vi "Insight LT.vi"(0 "Scroll Timing":i32=1500, 1 "ZONE \nCONFIGURATION":T1(ring), 2 "Digital Module":T2, 3 "Zone 4 Data":string[](array[string]), 4 "Zone 3 Data":string[](array[string]), 5 "Zone 2 Data":string[](array[string]), 6 "Zone 1 Data":string[](array[string])) -> ()   [LabVIEW 2012]
uses:
  <vilib>/Rock Robotics/SystemInterfaces/Typedef/FPGA_TypedefDigitalModule.ctl
panel:
  out "Zone 1 Index Count Line 2":i8
  out "Index Timer":dbl
  out "Zone 4 Index Count":i8
  out "Zone 3 Index Count":i8
  out "Zone 2 Index Count":i8
  out "Zone 1 Index Count":i8
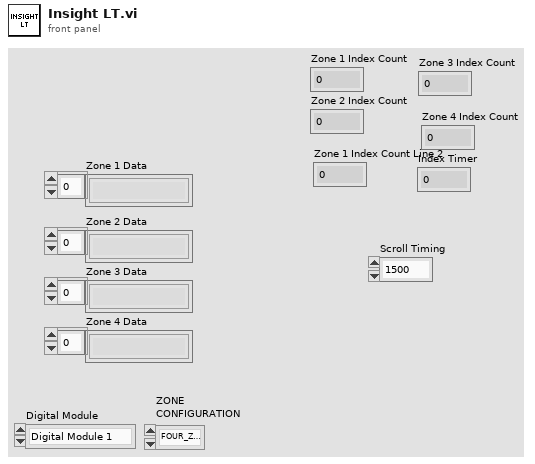
[diagram p1: front panel]
types:
  T1 = enum16{"FOUR_ZONES", "ONE_ZONE_TWO_LINES", "TWO_ZONES_ONE_LINE"}
  T2 = typedef "FPGA_TypedefDigitalModule.ctl" = enum16{"Digital Module 1", "Digital Module 2"}
  T3 = typedef "WPI_I2CDevRef.ctl" = cluster{"DevStatus":errorcluster, "Digital Module":T2, "Device Address":u8}
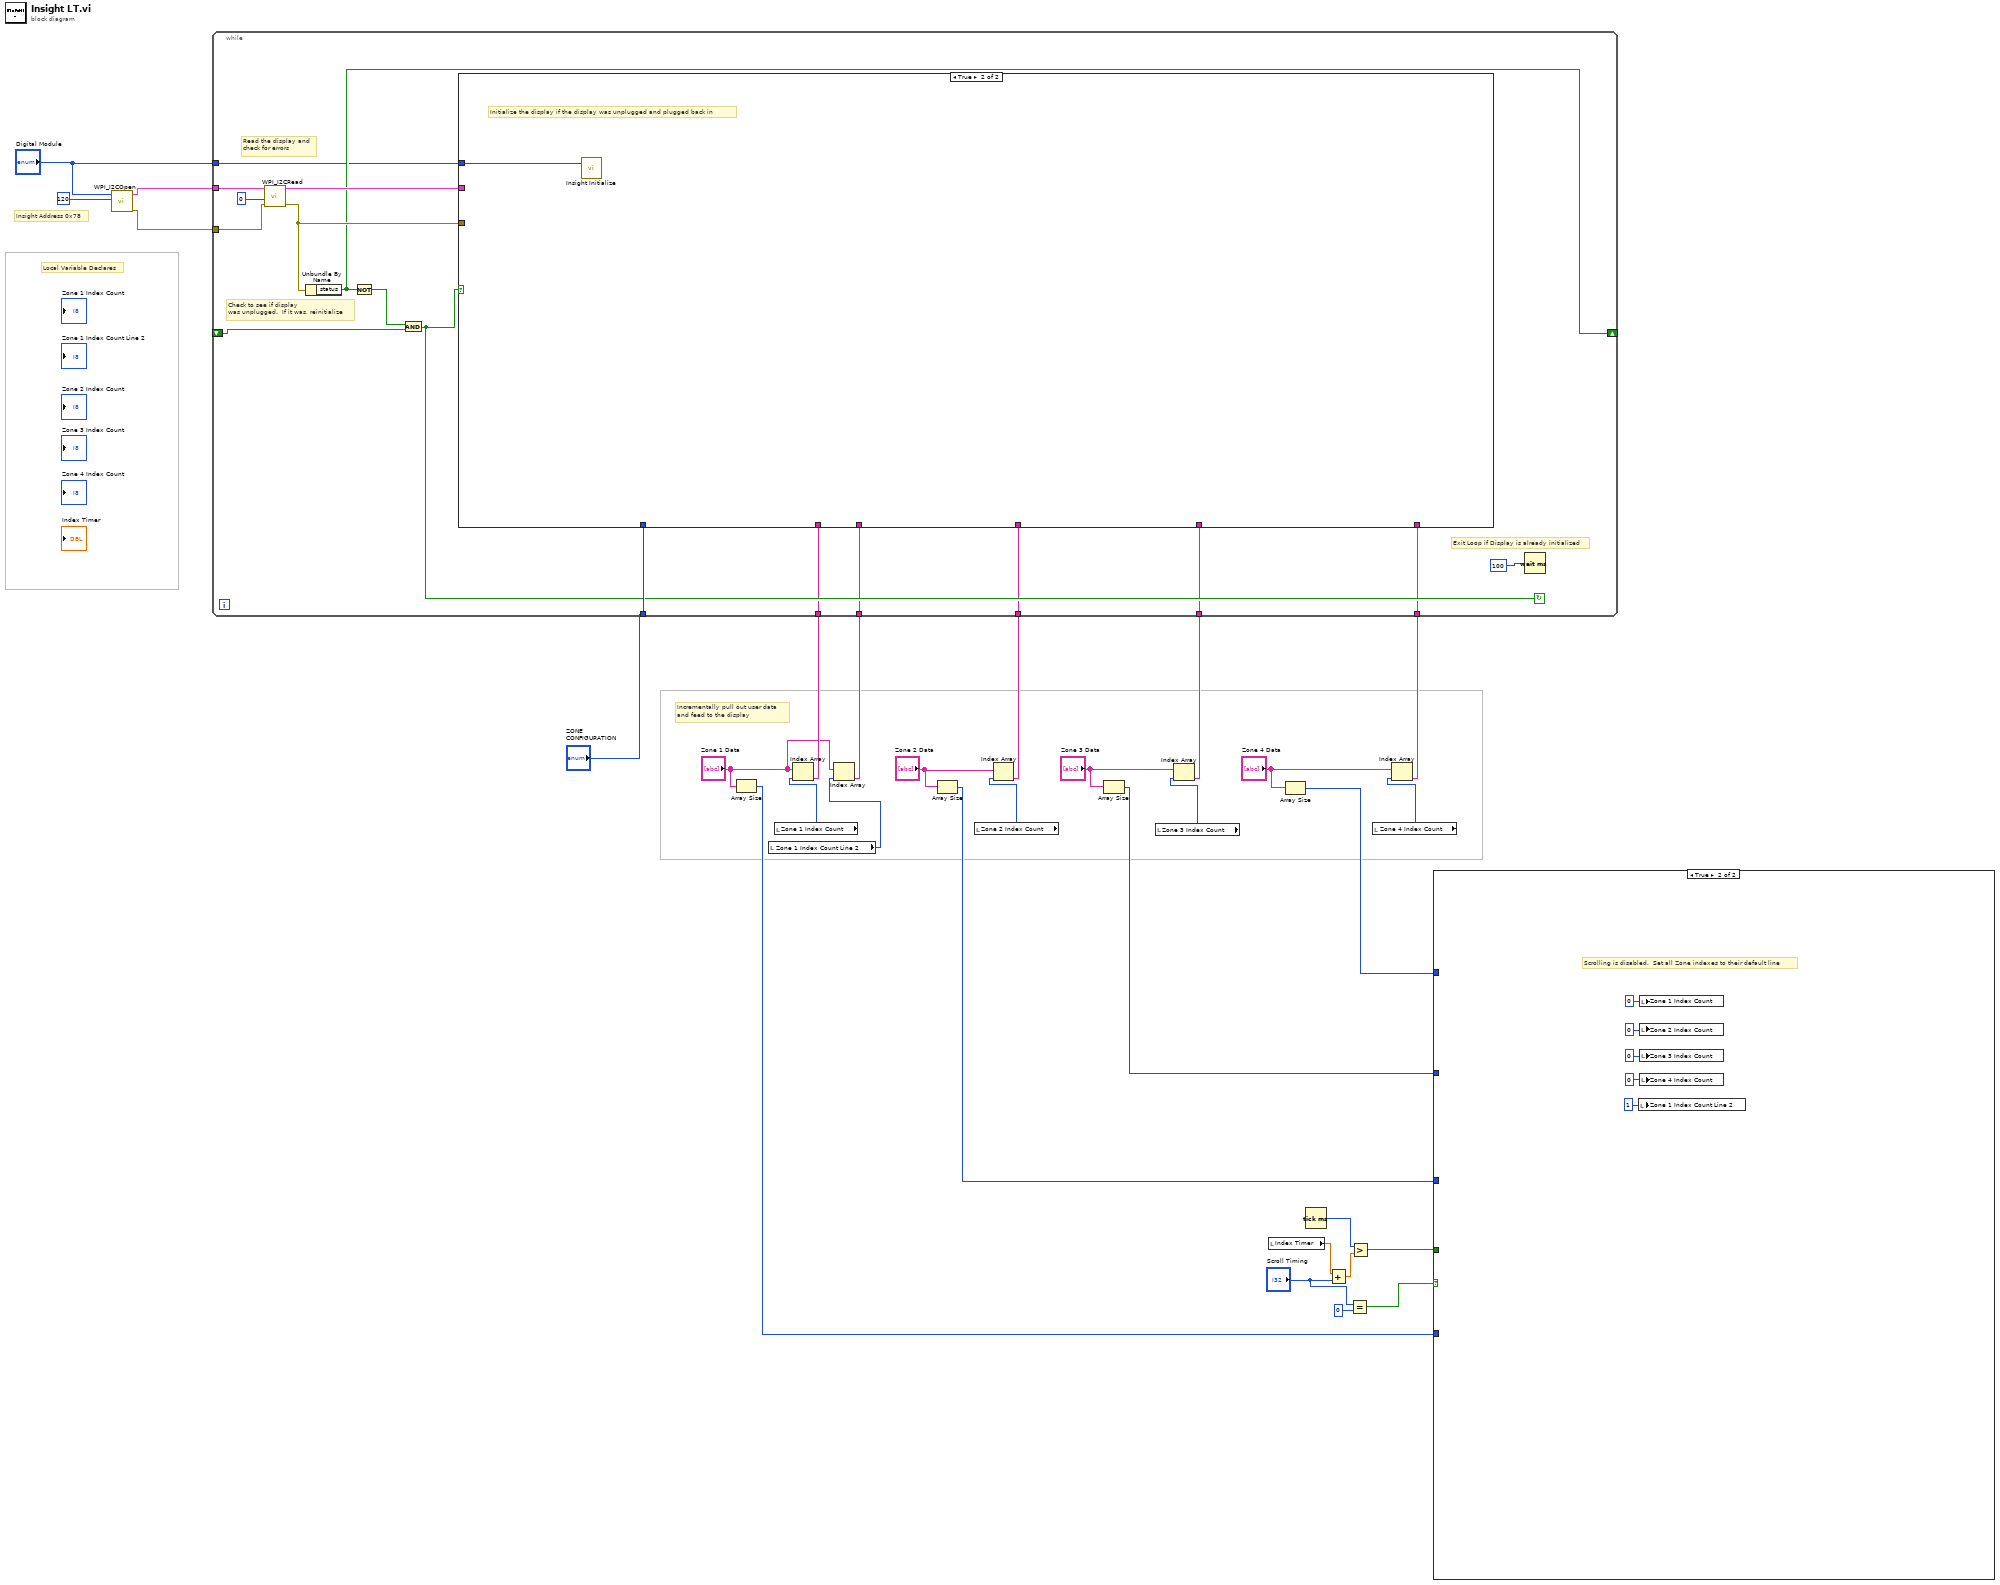
[diagram p0: block diagram]
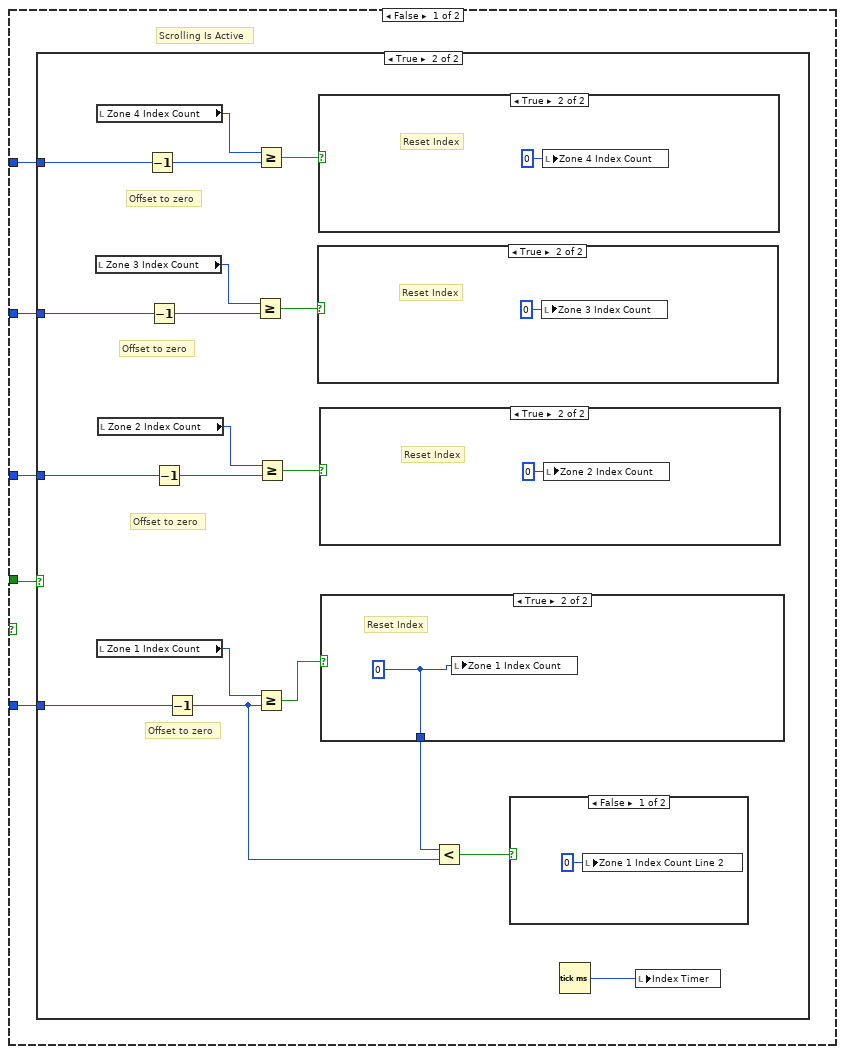
[diagram p2: hidden frame]
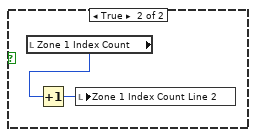
[diagram p4: hidden frame]
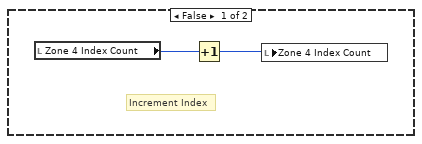
[diagram p5: hidden frame]
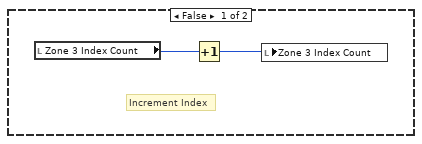
[diagram p6: hidden frame]
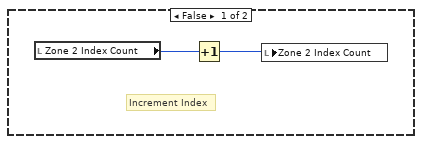
[diagram p7: hidden frame]
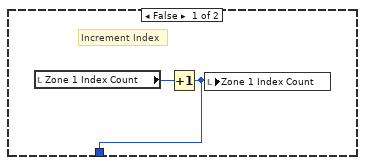
[diagram p8: hidden frame]
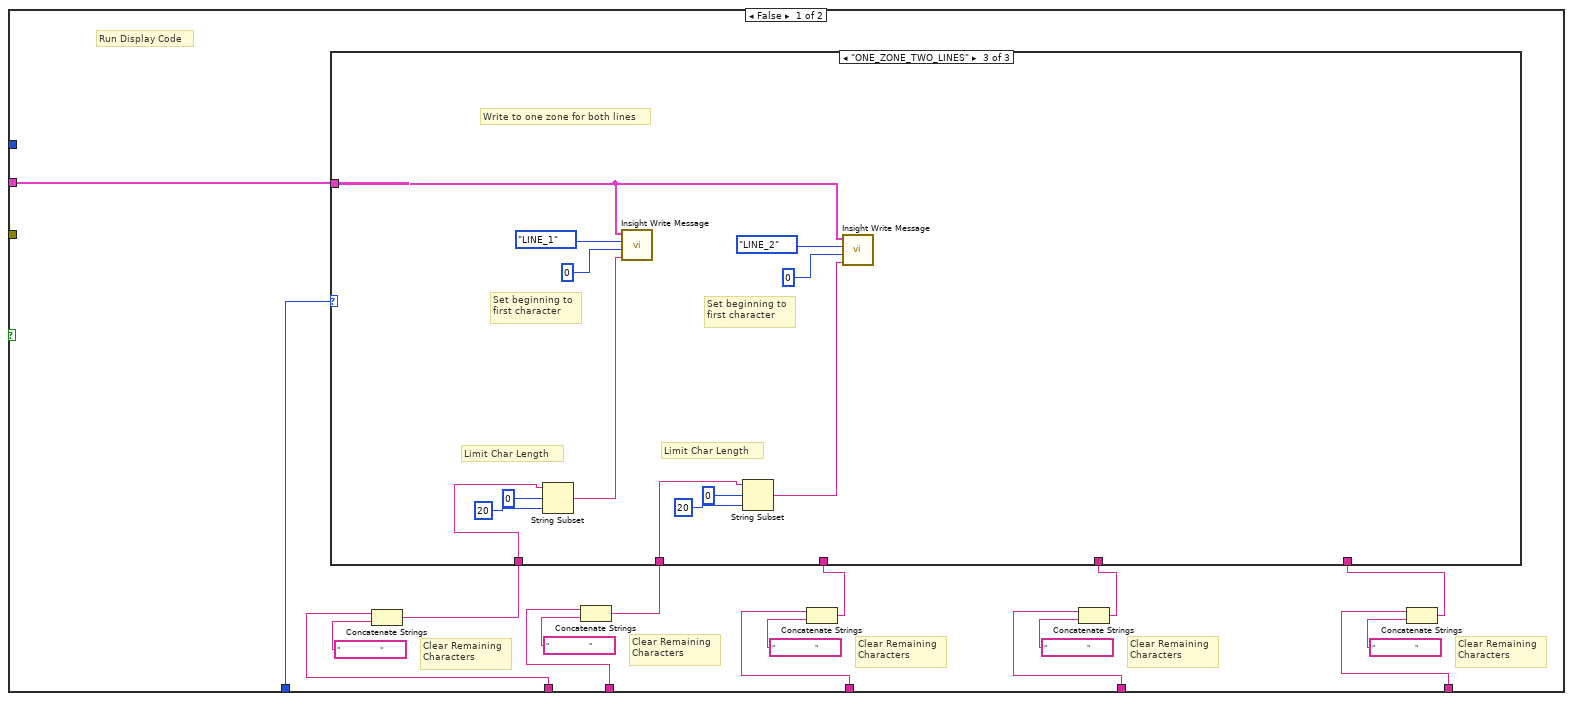
[diagram p9: hidden frame]
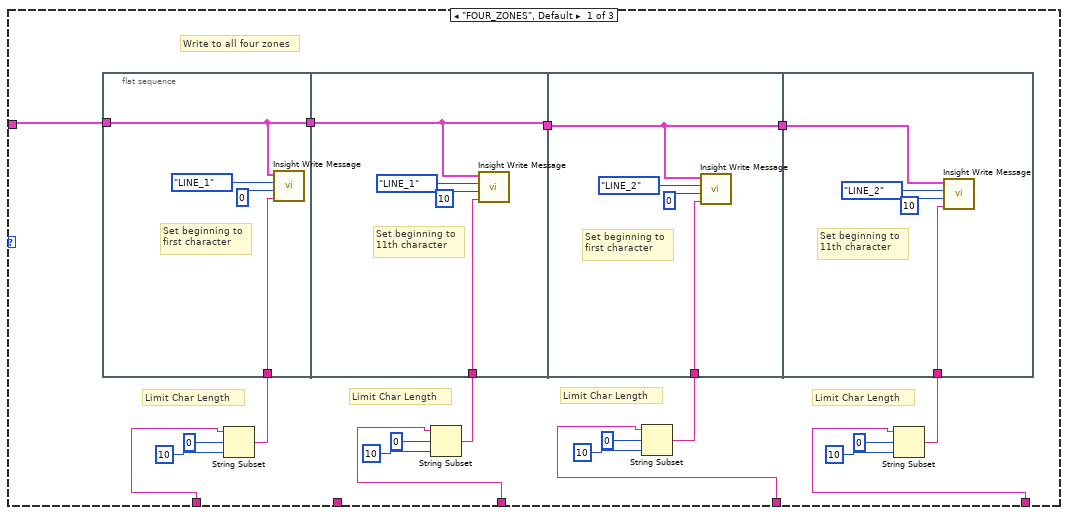
[diagram p10: hidden frame]
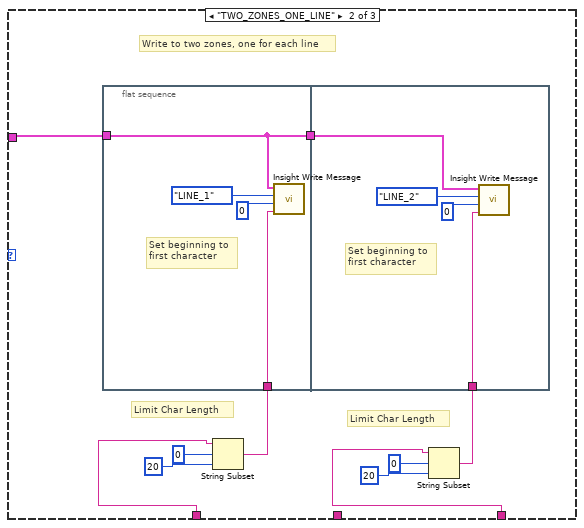
[diagram p11: hidden frame]
diagram:
  # "Incrementally pull out user data\nand feed to the display"
  # "Local Variable Declares"
  # "Insight Address 0x78"
  n1 = call <vilib>:"WPI_I2COpen.vi"("Device Address"=u8 120, "Digital Module (Module 1)"="Digital Module") -> ("error out"=w28:errorcluster, "I2CDevRef"=w29:T3)  [unwired: 8 in]
  n2 = Array Size(array="Zone 1 Data") -> (size(s)=w21:i32)
  n3 = local read "Zone 1 Index Count Line 2"() -> (w4:i8)
  n4 = local read "Zone 1 Index Count"() -> (w6:i8)
  n5 = Index Array(array="Zone 1 Data", index=w6) -> (element=w17:string)
  n6 = Index Array(array="Zone 1 Data", index=w4) -> (element=w5:string)
  n7 = Array Size(array="Zone 2 Data") -> (size(s)=w20:i32)
  n8 = local read "Zone 2 Index Count"() -> (w16:i8)
  n9 = Index Array(array="Zone 2 Data", index=w16) -> (element=w10:string)
  n10 = Array Size(array="Zone 3 Data") -> (size(s)=w19:i32)
  n11 = local read "Zone 3 Index Count"() -> (w15:i8)
  n12 = Index Array(array="Zone 3 Data", index=w15) -> (element=w9:string)
  n13 = local read "Index Timer"() -> (w24:dbl)
  n14 = Array Size(array="Zone 4 Data") -> (size(s)=w18:i32)
  n15 = Tick Count (ms)() -> (millisecond timer value=w25:u32)
  n16 = Add(x=w24, y="Scroll Timing") -> (x+y=w23:dbl)
  n17 = Equal?(x="Scroll Timing", y=i8 0) -> (x = y?=w3:bool)
  n18 = Greater?(x=w25, y=w23) -> (0:w22:bool)
  n19 = local read "Zone 4 Index Count"() -> (w14:i8)
  n20 = Index Array(array="Zone 4 Data", index=w14) -> (element=w8:string)
  n21 = while {
    shift-right: [w40] -> _
    shift-left: _ -> [w41]
    tunnel: w29 -> [w43]
    tunnel: w28 -> [w42]
    tunnel: "ZONE \nCONFIGURATION" -> [w38]
    tunnel: "Digital Module" -> [w36]
    tunnel: w17 -> [w35]
    tunnel: w10 -> [w34]
    tunnel: w9 -> [w33]
    tunnel: w8 -> [w32]
    tunnel: w5 -> [w31]
    stop <- w37 continue-if-true
    # "Read the display and\ncheck for errors"
    # "Exit Loop if Display is already initialized"
    # "Check to see if display\nwas unplugged.  If it was, reinitialize"
    n22 = call <vilib>:"WPI_I2CRead.vi"("error in (no error)"=w42, "I2CBytesToRead"=u8 0, "I2CDevRef"=w43) -> ("error out"=w44:errorcluster, "I2CDevRef"=w45:T3)  [unwired: 6 in, 1 out]
    n23 = Unbundle By Name(w44) -> ("status"=w40:bool)
    n24 = Not(x=w40) -> (.not. x?=w39:bool)
    n25 = And(x=w39, y=w41) -> (x .and. y?=w37:bool)
    n26 = case shown="True" w37 {
      tunnel: w45 -> [w63 _]
      tunnel: w44 -> [_ _]
      tunnel: w38 -> [w64 _]
      tunnel: w36 -> [_ w132]
      tunnel: w35 -> [w61 _]
      tunnel: w34 -> [w53 _]
      tunnel: w33 -> [w54 _]
      tunnel: w32 -> [w56 _]
      tunnel: w31 -> [w49 _]
      frame False {
        # "Clear Remaining\nCharacters"
        # "Clear Remaining\nCharacters"
        # "Clear Remaining\nCharacters"
        # "Clear Remaining\nCharacters"
        # "Clear Remaining\nCharacters"
        # "Run Display Code"
        n27 = Concatenate Strings(w61, "                    " ("string")) -> (w62:string)
        n28 = Concatenate Strings(w49, "                    " ("string")) -> (w48:string)
        n29 = Concatenate Strings(w53, "                    " ("string")) -> (w52:string)
        n30 = Concatenate Strings(w54, "                    " ("string")) -> (w51:string)
        n31 = Concatenate Strings(w56, "                    " ("string")) -> (w55:string)
        n32 = case shown="\"ONE_ZONE_TWO_LINES\"" w64 {
          tunnel: w63 -> [w84 w110 w123]
          tunnel: w62 -> [w68 w102 w126]
          tunnel: w52 -> [w67 w101 _]
          tunnel: w51 -> [w66 _ _]
          tunnel: w55 -> [w65 _ _]
          tunnel: w48 -> [_ _ w119]
          frame "FOUR_ZONES", Default {
            # "Write to all four zones"
            # "Limit Char Length"
            # "Limit Char Length"
            # "Limit Char Length"
            # "Limit Char Length"
            n33 = flat-sequence {
              tunnel: w84 -> [w86]
              tunnel: [w86] -> w83
              tunnel: w78 -> [w85]
              tunnel: w83 -> [w90]
              tunnel: [w90] -> w82
              tunnel: w75 -> [w89]
              tunnel: w82 -> [w94]
              tunnel: [w94] -> w81
              tunnel: w70 -> [w93]
              tunnel: w81 -> [w98]
              tunnel: w69 -> [w97]
              frame #0 {
                # "Set beginning to\nfirst character"
                n34 = call "Insight Write Message.vi"("User Data"=w85, "Position"=u8 0, "Line"=enum16{"LINE_1", "LINE_2"}."LINE_1", "I2CDevRef"=w86) -> ()  [unwired: 1 in]
              }
              frame #1 {
                # "Set beginning to\n11th character"
                n35 = call "Insight Write Message.vi"("User Data"=w89, "Position"=u8 10, "Line"=enum16{"LINE_1", "LINE_2"}."LINE_1", "I2CDevRef"=w90) -> ()  [unwired: 1 in]
              }
              frame #2 {
                # "Set beginning to\nfirst character"
                n36 = call "Insight Write Message.vi"("User Data"=w93, "Position"=u8 0, "Line"=enum16{"LINE_1", "LINE_2"}."LINE_2", "I2CDevRef"=w94) -> ()  [unwired: 1 in]
              }
              frame #3 {
                # "Set beginning to\n11th character"
                n37 = call "Insight Write Message.vi"("User Data"=w97, "Position"=u8 10, "Line"=enum16{"LINE_1", "LINE_2"}."LINE_2", "I2CDevRef"=w98) -> ()  [unwired: 1 in]
              }
            }
            n38 = String Subset(string=w68, offset (0)=0, length (rest)=10 ("length (rest)")) -> (substring=w78:string)
            n39 = String Subset(string=w67, offset (0)=0, length (rest)=10 ("length (rest)")) -> (substring=w75:string)
            n40 = String Subset(string=w66, offset (0)=0, length (rest)=10 ("length (rest)")) -> (substring=w70:string)
            n41 = String Subset(string=w65, offset (0)=0, length (rest)=10 ("length (rest)")) -> (substring=w69:string)
          }
          frame "TWO_ZONES_ONE_LINE" {
            # "Write to two zones, one for each line"
            # "Limit Char Length"
            # "Limit Char Length"
            n42 = flat-sequence {
              tunnel: w110 -> [w112]
              tunnel: [w112] -> w109
              tunnel: w103 -> [w111]
              tunnel: w109 -> [w116]
              tunnel: w104 -> [w115]
              frame #0 {
                # "Set beginning to\nfirst character"
                n43 = call "Insight Write Message.vi"("User Data"=w111, "Position"=u8 0, "Line"=enum16{"LINE_1", "LINE_2"}."LINE_1", "I2CDevRef"=w112) -> ()  [unwired: 1 in]
              }
              frame #1 {
                # "Set beginning to\nfirst character"
                n44 = call "Insight Write Message.vi"("User Data"=w115, "Position"=u8 0, "Line"=enum16{"LINE_1", "LINE_2"}."LINE_2", "I2CDevRef"=w116) -> ()  [unwired: 1 in]
              }
            }
            n45 = String Subset(string=w102, offset (0)=0, length (rest)=20 ("length (rest)")) -> (substring=w103:string)
            n46 = String Subset(string=w101, offset (0)=0, length (rest)=20 ("length (rest)")) -> (substring=w104:string)
          }
          frame "ONE_ZONE_TWO_LINES" {
            # "Set beginning to\nfirst character"
            # "Set beginning to\nfirst character"
            # "Write to one zone for both lines"
            # "Limit Char Length"
            # "Limit Char Length"
            n47 = String Subset(string=w126, offset (0)=0, length (rest)=20 ("length (rest)")) -> (substring=w127:string)
            n48 = call "Insight Write Message.vi"("User Data"=w127, "Position"=u8 0, "Line"=enum16{"LINE_1", "LINE_2"}."LINE_1", "I2CDevRef"=w123) -> ()  [unwired: 1 in]
            n49 = String Subset(string=w119, offset (0)=0, length (rest)=20 ("length (rest)")) -> (substring=w120:string)
            n50 = call "Insight Write Message.vi"("User Data"=w120, "Position"=u8 0, "Line"=enum16{"LINE_1", "LINE_2"}."LINE_2", "I2CDevRef"=w123) -> ()  [unwired: 1 in]
          }
        }
      }
      frame True {
        # "Initialize the display if the display was unplugged and plugged back in"
        n51 = call "Insight Initialize.vi"("Digital Module"=w132) -> ()  [unwired: 2 in]
      }
    }
    n52 = Wait (ms)(milliseconds to wait=u32 100) -> ()  [unwired: 1 out]
  }
  n53 = case shown="True" w3 {
    tunnel: w22 -> [w137 _]
    tunnel: w21 -> [w136 _]
    tunnel: w20 -> [w135 _]
    tunnel: w19 -> [w134 _]
    tunnel: w18 -> [w133 _]
    frame False {
      # "Scrolling Is Active"
      n54 = case shown="True" w137 {
        tunnel: w136 -> [_ w148]
        tunnel: w135 -> [_ w145]
        tunnel: w134 -> [_ w146]
        tunnel: w133 -> [_ w147]
        frame False {
          # "Do Not Index the Zone Counters"
        }
        frame True {
          # "Offset to zero"
          # "Offset to zero"
          # "Offset to zero"
          # "Offset to zero"
          n55 = local read "Zone 3 Index Count"() -> (w151:i8)
          n56 = local read "Zone 4 Index Count"() -> (w150:i8)
          n57 = local read "Zone 1 Index Count"() -> (w141:i8)
          n58 = local read "Zone 2 Index Count"() -> (w154:i8)
          n59 = Decrement(x=w147) -> (x-1=w142:i32)
          n60 = Decrement(x=w146) -> (x-1=w143:i32)
          n61 = Decrement(x=w145) -> (x-1=w144:i32)
          n62 = Decrement(x=w148) -> (x-1=w139:i32)
          n63 = Greater Or Equal?(x=w151, y=w143) -> (x >= y?=w152:bool)
          n64 = Greater Or Equal?(x=w150, y=w142) -> (x >= y?=w149:bool)
          n65 = Greater Or Equal?(x=w141, y=w139) -> (x >= y?=w155:bool)
          n66 = Greater Or Equal?(x=w154, y=w144) -> (x >= y?=w153:bool)
          n67 = case shown="True" w152 {
            frame False {
              # "Increment Index"
              n68 = local read "Zone 3 Index Count"() -> (w164:i8)
              n69 = Increment(x=w164) -> (x+1=w163:i8)
              n70 = local write "Zone 3 Index Count"(w163) -> ()
            }
            frame True {
              # "Reset Index"
              n71 = local write "Zone 3 Index Count"(i8 0 ("Zone 1 Index Count")) -> ()
            }
          }
          n72 = case shown="True" w149 {
            frame False {
              # "Increment Index"
              n73 = local read "Zone 4 Index Count"() -> (w161:i8)
              n74 = Increment(x=w161) -> (x+1=w160:i8)
              n75 = local write "Zone 4 Index Count"(w160) -> ()
            }
            frame True {
              # "Reset Index"
              n76 = local write "Zone 4 Index Count"(i8 0 ("Zone 1 Index Count")) -> ()
            }
          }
          n77 = case shown="True" w153 {
            frame False {
              # "Increment Index"
              n78 = local read "Zone 2 Index Count"() -> (w167:i8)
              n79 = Increment(x=w167) -> (x+1=w166:i8)
              n80 = local write "Zone 2 Index Count"(w166) -> ()
            }
            frame True {
              # "Reset Index"
              n81 = local write "Zone 2 Index Count"(i8 0 ("Zone 1 Index Count")) -> ()
            }
          }
          n82 = case shown="True" w155 {
            tunnel: [w169 w171] -> w138
            frame False {
              # "Increment Index"
              n83 = local read "Zone 1 Index Count"() -> (w170:i8)
              n84 = Increment(x=w170) -> (x+1=w169:i8)
              n85 = local write "Zone 1 Index Count"(w169) -> ()
            }
            frame True {
              w171 = i8 0 ("Zone 1 Index Count")
              # "Reset Index"
              n86 = local write "Zone 1 Index Count"(w171) -> ()
            }
          }
          n87 = Less?(x=w138, y=w139) -> (x < y?=w140:bool)
          n88 = case shown="False" w140 {
            frame False {
              n89 = local write "Zone 1 Index Count Line 2"(i8 0 ("Zone 1 Index Count Line 2")) -> ()
            }
            frame True {
              n90 = local read "Zone 1 Index Count"() -> (w158:i8)
              n91 = Increment(x=w158) -> (x+1=w159:i8)
              n92 = local write "Zone 1 Index Count Line 2"(w159) -> ()
            }
          }
          n93 = Tick Count (ms)() -> (millisecond timer value=w156:u32)
          n94 = local write "Index Timer"(w156) -> ()
        }
      }
    }
    frame True {
      # "Scrolling is disabled.  Set all Zone indexes to their default line"
      n95 = local write "Zone 1 Index Count Line 2"(i8 1 ("Zone 4 Index Count")) -> ()
      n96 = local write "Zone 1 Index Count"(i8 0 ("Zone 4 Index Count")) -> ()
      n97 = local write "Zone 2 Index Count"(i8 0 ("Zone 4 Index Count")) -> ()
      n98 = local write "Zone 3 Index Count"(i8 0 ("Zone 4 Index Count")) -> ()
      n99 = local write "Zone 4 Index Count"(i8 0 ("Zone 4 Index Count")) -> ()
    }
  }
